vi "Run 4.vi"(11 "NXT/EV3":T1) -> (3 "EV3 out":T1)   [LabVIEW 2016]
uses:
  <vilib>/NXT/Subs/LVHSConnector.ctl
  <vilib>/NXT/LegoClasses/BrickReference/BrickReference.lvclass
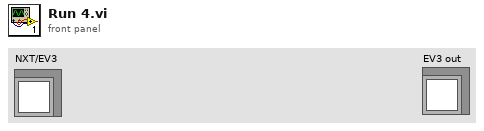
[diagram p1: front panel]
types:
  T1 = typedef "LVHSConnector.ctl" = refnum<class "BrickReference.lvclass">
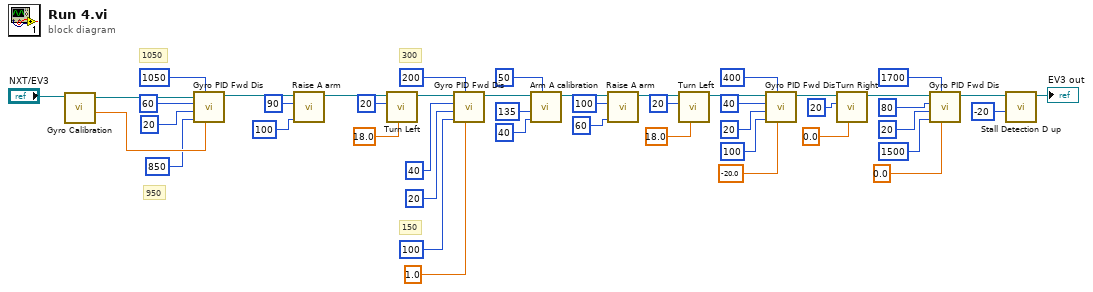
[diagram p0: block diagram]
diagram:
  # "950"
  # "1050"
  # "150"
  # "300"
  n1 = call "Gyro Calibration.vi"("NXT/EV3"="NXT/EV3") -> ("Degrees"=w45:sgl, "NXT/EV3"=w1:T1)  [unwired: 6 in, 1 out]
  n2 = call "Gyro PID Fwd Dis.vi"("Target angle"=w45, "Threshold to stop"=1050, "Threshold to slow"=850, "Min. speed"=20, "Max. speed"=60, "EV3 in"=w1) -> ("EV3 out"=w47:T1)  [unwired: 5 in]
  n3 = call "Raise A arm.vi"("Power"=i8 100, "Rotation"=90, "EV3 in"=w47) -> ("EV3 out"=w30:T1)  [unwired: 8 in]
  n4 = call "Turn Left.vi"("Turning angle"=sgl 18.0, "Motor B (right)"=i8 20, "EV3 in"=w30) -> ("EV3 out"=w29:T1)  [unwired: 8 in]
  n5 = call "Gyro PID Fwd Dis.vi"("Target angle"=sgl 1.0, "Threshold to stop"=200, "Threshold to slow"=100, "Min. speed"=20, "Max. speed"=40, "EV3 in"=w29) -> ("EV3 out"=w28:T1)  [unwired: 5 in]
  n6 = call "Arm A calibration.vi"("Cali. Power"=i8 50, "Down Power"=i8 40, "Rotation"=135, "NXT/EV3"=w28) -> ("NXT/EV3"=w24:T1)  [unwired: 7 in]
  n7 = call "Raise A arm.vi"("Power"=i8 60, "Rotation"=100, "EV3 in"=w24) -> ("EV3 out"=w21:T1)  [unwired: 8 in]
  n8 = call "Turn Left.vi"("Turning angle"=sgl 18.0, "Motor B (right)"=i8 20, "EV3 in"=w21) -> ("EV3 out"=w16:T1)  [unwired: 8 in]
  n9 = call "Gyro PID Fwd Dis.vi"("Target angle"=sgl -20.0, "Threshold to stop"=400, "Threshold to slow"=100, "Min. speed"=20, "Max. speed"=40, "EV3 in"=w16) -> ("EV3 out"=w14:T1)  [unwired: 5 in]
  n10 = call "Turn Right.vi"("Turning angle"=sgl 0.0, "Motor B (right)"=i8 20, "EV3 in"=w14) -> ("EV3 out"=w6:T1)  [unwired: 8 in]
  n11 = call "Gyro PID Fwd Dis.vi"("Target angle"=sgl 0.0, "Threshold to stop"=1700, "Threshold to slow"=1500, "Min. speed"=20, "Max. speed"=80, "EV3 in"=w6) -> ("EV3 out"=w5:T1)  [unwired: 5 in]
  n12 = call "Stall Detection D up.vi"("Power"=i8 -20, "NXT/EV3"=w5) -> ("NXT/EV3"=→"EV3 out":T1)  [unwired: 9 in]
